vi "check.vi"(9 "input result":bool, 10 "input string":string) -> (0 "Array":bool[](array[boolean]), 1 "Result":bool, 2 "parameter value":string, 3 "function value":string)   [LabVIEW 2017]
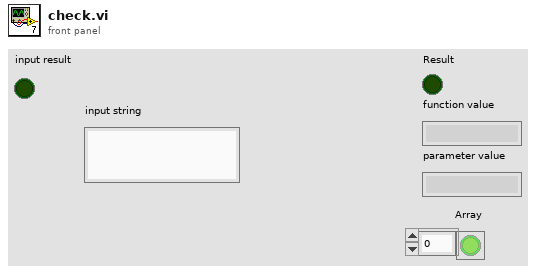
[diagram p1: front panel]
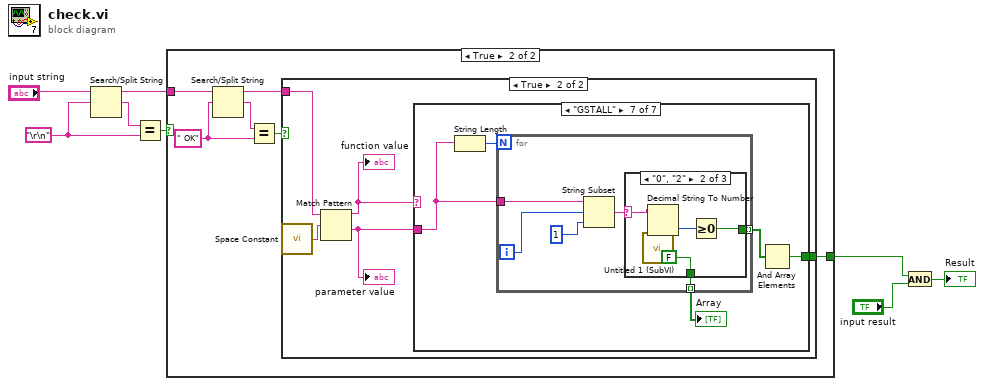
[diagram p0: block diagram]
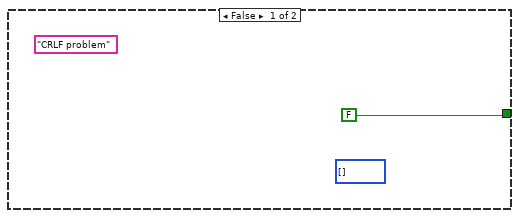
[diagram p2: hidden frame]
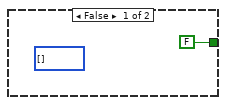
[diagram p3: hidden frame]
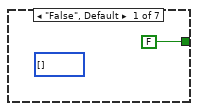
[diagram p4: hidden frame]
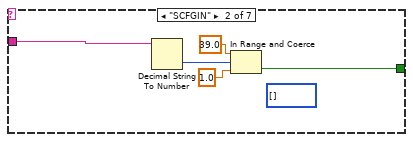
[diagram p5: hidden frame]
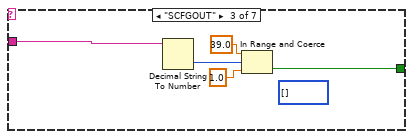
[diagram p6: hidden frame]
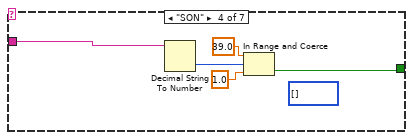
[diagram p7: hidden frame]
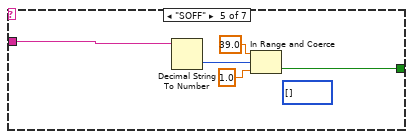
[diagram p8: hidden frame]
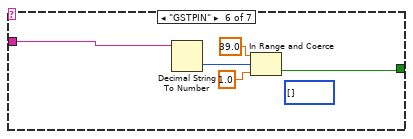
[diagram p9: hidden frame]
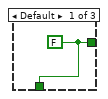
[diagram p10: hidden frame]
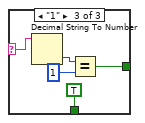
[diagram p11: hidden frame]
diagram:
  w4 = "\r\n"
  n1 = Search/Split String(string="input string", search string/char (-)=w4) -> (substring before match=w7:string, match + rest of string=w5:string)  [unwired: 1 in, 1 out]
  n2 = Equal?(x=w5, y=w4) -> (x = y?=w6:bool)
  n3 = case shown="True" w6 {
    tunnel: w7 -> [_ w15]
    tunnel: [FALSE ("Boolean") w10] -> w3
    frame False {
      (unwired) i32[] [] ("Numeric")
      (unwired) "CRLF problem"
    }
    frame True {
      w13 = " OK"
      n4 = Search/Split String(string=w15, search string/char (-)=w13) -> (substring before match=w11:string, match + rest of string=w14:string)  [unwired: 1 in, 1 out]
      n5 = Equal?(x=w14, y=w13) -> (x = y?=w12:bool)
      n6 = case shown="True" w12 {
        tunnel: w11 -> [_ w19]
        tunnel: [FALSE ("Boolean") w21] -> w10
        frame False {
          (unwired) i32[] [] ("Numeric")
        }
        frame True {
          n7 = call <vilib>:"Space Constant.vi"() -> ("String"=w20:string)
          n8 = Match Pattern(string=w19, regular expression=w20) -> (before substring=w18:string, after substring=w17:string)  [unwired: 1 in, 2 out]
          "function value" <- w18
          "parameter value" <- w17
          n9 = case shown="\"GSTALL\"" w18 {
            tunnel: [FALSE ("Boolean") w24 w29 w34 w39 w44 w50] -> w21
            tunnel: w17 -> [_ w23 w28 w33 w38 w43 w49]
            frame "False", Default {
              (unwired) i32[] [] ("Numeric")
            }
            frame "SCFGIN" {
              (unwired) i32[] [] ("Numeric")
              n10 = Decimal String To Number(string=w23) -> (number=w25:i32)  [unwired: 2 in, 1 out]
              n11 = In Range and Coerce(upper limit=39.0, x=w25, lower limit=1.0) -> (In Range?=w24:bool)  [unwired: 1 out]
            }
            frame "SCFGOUT" {
              (unwired) i32[] [] ("Numeric")
              n12 = Decimal String To Number(string=w28) -> (number=w30:i32)  [unwired: 2 in, 1 out]
              n13 = In Range and Coerce(upper limit=39.0, x=w30, lower limit=1.0) -> (In Range?=w29:bool)  [unwired: 1 out]
            }
            frame "SON" {
              (unwired) i32[] [] ("Numeric")
              n14 = Decimal String To Number(string=w33) -> (number=w35:i32)  [unwired: 2 in, 1 out]
              n15 = In Range and Coerce(upper limit=39.0, x=w35, lower limit=1.0) -> (In Range?=w34:bool)  [unwired: 1 out]
            }
            frame "SOFF" {
              (unwired) i32[] [] ("Numeric")
              n16 = Decimal String To Number(string=w38) -> (number=w40:i32)  [unwired: 2 in, 1 out]
              n17 = In Range and Coerce(upper limit=39.0, x=w40, lower limit=1.0) -> (In Range?=w39:bool)  [unwired: 1 out]
            }
            frame "GSTPIN" {
              (unwired) i32[] []
              n18 = Decimal String To Number(string=w43) -> (number=w45:i32)  [unwired: 2 in, 1 out]
              n19 = In Range and Coerce(upper limit=39.0, x=w45, lower limit=1.0) -> (In Range?=w44:bool)  [unwired: 1 out]
            }
            frame "GSTALL" {
              n20 = String Length(string=w49) -> (length=w52:i32)
              n21 = for {
                N: w52 -> [_]
                tunnel: w49 -> [w58]
                tunnel: [w57] -> w51 mode=indexing
                tunnel: [w53] -> w48 mode=indexing
                i -> [w54]
                n22 = String Subset(string=w58, offset (0)=w54, length (rest)=1 ("x")) -> (substring=w55:string)
                n23 = case shown="\"0\", \"2\"" w55 {
                  selector: w55 -> [_ w61 w68]
                  tunnel: [w59 w63 w65] -> w57
                  tunnel: [w59 FALSE TRUE] -> w53
                  frame Default {
                    w59 = FALSE ("Boolean")
                  }
                  frame "0", "2" {
                    n24 = Decimal String To Number(string=w61) -> (number=w62:i32)  [unwired: 2 in, 1 out]
                    n25 = Greater Or Equal To 0?(x=w62) -> (x >= 0?=w63:bool)
                  }
                  frame "1" {
                    n26 = Decimal String To Number(string=w68) -> (number=w67:i32)  [unwired: 2 in, 1 out]
                    n27 = Equal?(x=w67, y=1) -> (x = y?=w65:bool)
                  }
                }
              }
              "Array" <- w48
              n28 = call "Untitled 1 (SubVI).vi"() -> ()  [unwired: 12 in]
              n29 = And Array Elements(Boolean array=w51) -> (logical AND=w50:bool)
            }
          }
        }
      }
    }
  }
  n30 = And(x=w3, y="input result") -> (x .and. y?=→"Result":bool)
